vi "Find File Path.vi"(8 "error in":errorcluster, 10 "Filename":string, 11 "Configuration in":refnum<class "Configuration.lvclass">) -> (0 "error out":errorcluster, 2 "File Path":path, 3 "Configuration out":refnum<class "Configuration.lvclass">)   [LabVIEW 2018, in "Configuration.lvlib" / "Configuration.lvclass"]
doc: "This program locates the path to the config.ini file associated with the test station in which it is deployed. \n\nIt does this by using the application path reference and searches up a directory recursively until it locates a file named config.ini. \n\nIt is imperative to format the file structure as defined in the coding convention for this reason."
uses:
  Configuration.lvclass
  Configuration.lvclass/Configuration.ctl
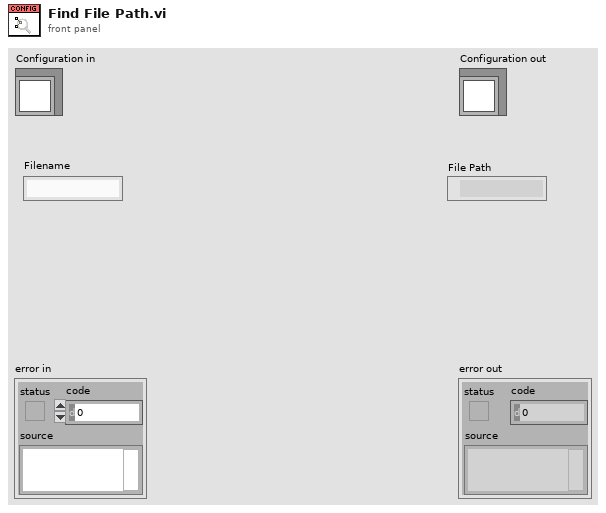
[diagram p1: front panel]
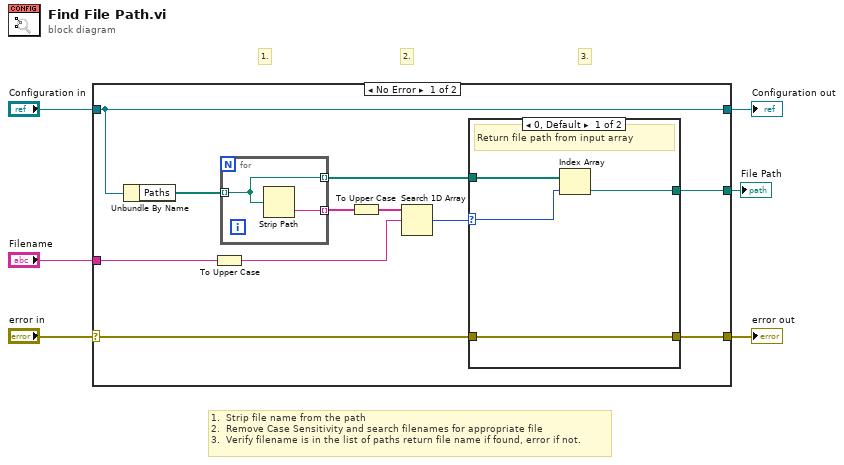
[diagram p0: block diagram]
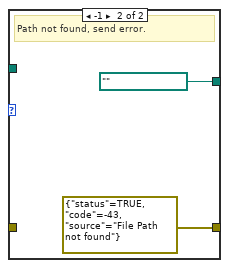
[diagram p2: hidden frame]
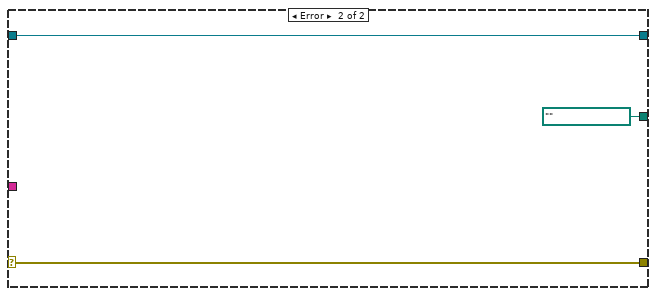
[diagram p3: hidden frame]
diagram:
  # "1.  Strip file name from the path\n2.  Remove Case Sensitivity and search filenames for appropriate file\n3.  Verify filename is in the list of paths return file name if found, error if not."
  # "3."
  # "2."
  # "1."
  n1 = case shown="No Error" "error in" {
    selector: "error in" -> [w15 w28]
    tunnel: [w11 w28] -> w5
    tunnel: [w8 w27] -> w3
    tunnel: "Configuration in" -> [w8 w27]
    tunnel: "Filename" -> [w16 _]
    tunnel: [w12 path "" ("Path")] -> w1
    frame No Error {
      n2 = Unbundle By Name(w8) -> ("Paths"=w7:path[])
      n3 = To Upper Case(1:w16) -> (0:w10:string)
      n4 = for {
        tunnel: w7 -> [w24] mode=indexing
        tunnel: [w25] -> w17 mode=indexing
        tunnel: [w24] -> w13 mode=indexing
        n5 = Strip Path(path=w24) -> (name=w25:string)  [unwired: 1 out]
      }
      n6 = To Upper Case(1:w17) -> (0:w9:string[])
      n7 = Search 1D Array(1D array=w9, element=w10) -> (index of element=w14:i32)  [unwired: 1 in]
      n8 = case shown="0, Default" w14 {
        selector: w14 -> [w20 _]
        tunnel: w15 -> [w18 _]
        tunnel: w13 -> [w21 _]
        tunnel: [w19 path "" ("Path")] -> w12
        tunnel: [w18 errorcluster {"status"=TRUE, "code"=-43, "source"="File Path not found"} ("error IO")] -> w11
        frame 0, Default {
          # "Return file path from input array"
          n9 = Index Array(array=w21, index=w20) -> (element=w19:path)
        }
        frame -1 {
          # "Path not found, send error."
        }
      }
    }
    frame Error {
    }
  }
  "error out" <- w5
  "Configuration out" <- w3
  "File Path" <- w1
